vi "Decode and Forward Message.vi"(8 "error in (no error)":errorcluster, 10 "Message undecoded":string, 11 "TCP Listener in":refnum<class "TCP Listener.lvclass">) -> (0 "error out":errorcluster, 3 "TCP Listener out":refnum<class "TCP Listener.lvclass">)   [LabVIEW 2026, in "TALOS.lvlib" / "TCP Listener.lvlib" / "TCP Listener.lvclass"]
uses:
  TCP Listener.lvclass
  C:/LabVIEW Code/TALOS/talos/Father of all uServices/Father of all uServices/Father of all uServices.lvclass
  C:/LabVIEW Code/TALOS/builds/Actor Framework PPL/Actor Framework.lvlibp/1abvi3w/vi.lib/ActorFramework/Actor/Actor.lvclass
  Guardian/Guardian Messages/Message to uService Msg/Message to uService Msg.lvclass/Message to uService Msg.ctl
  Ancestor/Ancestor/Ancestor.lvclass/Ancestor.ctl
  Guardian/Guardian Messages/TCP-SV Message Interpreter Msg/TCP-SV Message Interpreter Msg.lvclass/TCP-SV Message Interpreter Msg.ctl
  Father of all uServices/Father of all uServices/Father of all uServices.lvclass/Father of all uServices.ctl
  TCP Listener.lvclass/TCP Listener.ctl
  Guardian/Guardian Messages/Message to uService Msg/Send Message to uService.vi
  Father of all uServices/Father of all uServices/Children Methods/Update GUI.vi
  Support VIs/Generate Error.vi
  FGV/Error Memory/Get Error Description.vi
  Support VIs/Get PC name.vi
  Ancestor/Ancestor/Read ID.vi
  Support VIs/Get Class Name.vi
  FGV/Error Memory/Error Memory Core.vi
  <vilib>/AdvancedString/Delimited String to 1D String Array.vi
  <vilib>/AdvancedString/Delimited String to 1D String Array (string).vi
  Support VIs/Circus Root Path.vi
  FGV/Error Memory/Error Crt Lvl checker.vi
  FGV/Error Memory/Error Memory Core.vi/40c8088d-b597-4017-91af-faa98e00292e.vi
  FGV/Error Memory/Error Memory Core.vi/d4a3ab98-063c-4e44-b43d-fbdcfe6c2be2.vi
  Father of all uServices/Father of all uServices/Father of all uServices.lvclass
  builds/Actor Framework PPL/Actor Framework.lvlibp/1abvi3w/vi.lib/ActorFramework/Message Enqueuer/Enqueue.vi
  Support VIs/Global Memory.vi
  <vilib>/Utility/LVClass/Get LV Class Name.vi
  Support VIs/Is in Packed Library.vi
  Support VIs/TALOS Root path.vi
  Support VIs/Read CSV worksheet.vi
  Support VIs/Global Constants.vi
  <vilib>/Utility/error.llb/General Error Handler.vi
  Support VIs/Error Log.vi
  Father of all uServices/Father of all uServices/Children Methods/Get GUI Item Value - String.vi
  Father of all uServices/Father of all uServices/Multiline string updater.vi
  Guardian/Guardian Messages/Message to uService Msg/Message to uService Msg.lvclass
  Ancestor/Ancestor/Ancestor.lvclass
  <vilib>/Comparison/Equal/Equal Functor/Equal Functor.lvclass
  Guardian/Guardian Messages/TCP-SV Message Interpreter Msg/TCP-SV Message Interpreter Msg.lvclass
  builds/Actor Framework PPL/Actor Framework.lvlibp/1abvi3w/vi.lib/ActorFramework/Actor/Actor.lvclass
  TALOS.lvlib
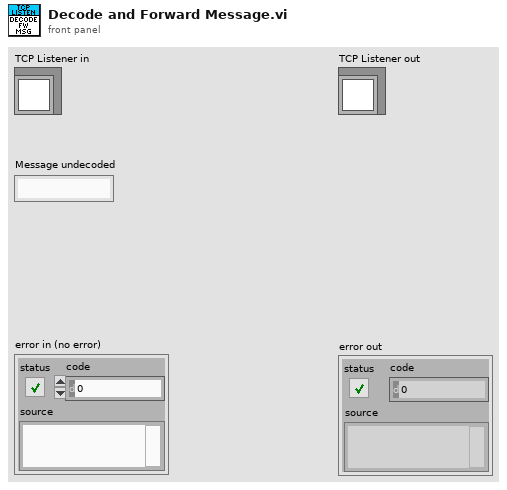
[diagram p1: front panel]
types:
  T1 = typedef "TALOS.lvlib/TCP Writer.lvlib/TCP Writer.lvclass/TCP Message Internal Composition.ctl" = cluster{"uS/GD ID":string, "Message":string, "Data":variant}
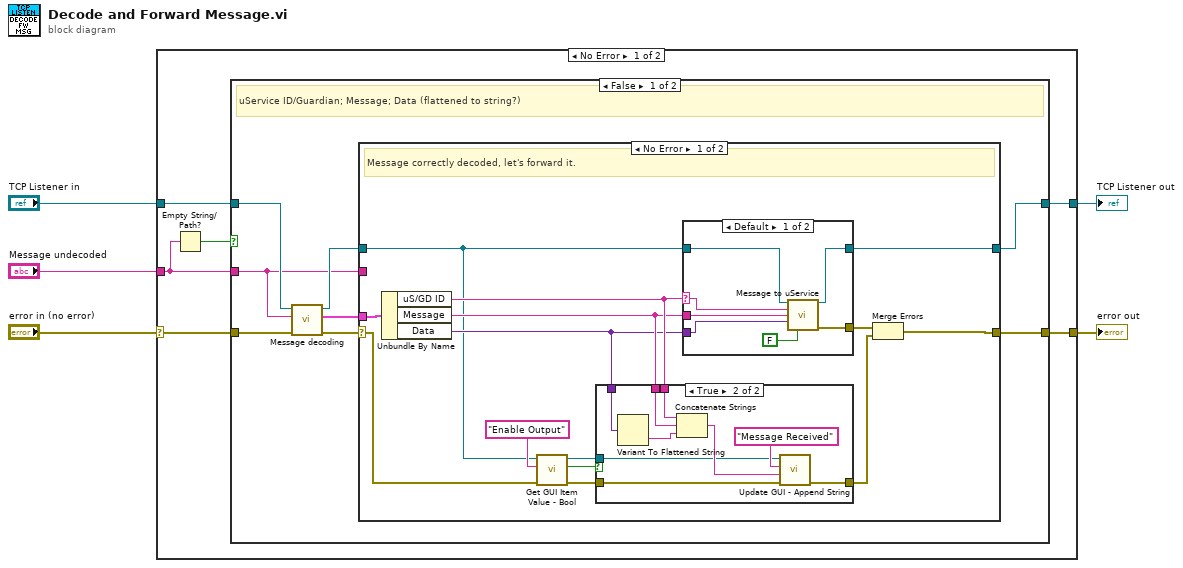
[diagram p0: block diagram]
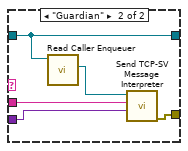
[diagram p3: hidden frame]
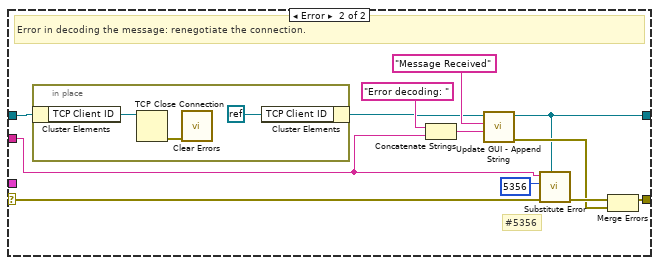
[diagram p4: hidden frame]
diagram:
  n1 = case shown="No Error" "error in (no error)" {
    selector: "error in (no error)" -> [w6 w73]
    tunnel: [w11 w73] -> w5
    tunnel: "TCP Listener in" -> [w10 w74]
    tunnel: [w9 w74] -> w3
    tunnel: "Message undecoded" -> [w8 _]
    frame No Error {
      n2 = Empty String/Path?(string/path=w8) -> (empty?=w7:bool)
      n3 = case shown="False" w7 {
        tunnel: w8 -> [w15 _]
        tunnel: w10 -> [w19 w72]
        tunnel: [w14 w72] -> w9
        tunnel: [w13 w71] -> w11
        tunnel: w6 -> [w12 w71]
        frame False {
          # "uService ID/Guardian; Message; Data (flattened to string?)"
          n4 = call-dynamic "Message decoding.vi"("error in (no error)"=w12, "Message"=w15, "TCP Listener in"=w19) -> ("error out"=w16:errorcluster, "Message decoded"=w18:T1, "TCP Listener out"=w17:refnum<class "TCP Listener.lvclass">)  [unwired: 6 in]
          n5 = case shown="No Error" w16 {
            selector: w16 -> [w24 w67]
            tunnel: w18 -> [w32 _]
            tunnel: [w28 w63] -> w13
            tunnel: w17 -> [w21 w61]
            tunnel: [w26 w56] -> w14
            tunnel: w15 -> [_ w64]
            frame No Error {
              # "Message correctly decoded, let's forward it."
              n6 = Unbundle By Name(w32) -> ("uS/GD ID"=w31:string, "Message"=w30:string, "Data"=w29:variant)
              n7 = call "Get GUI Item Value - Bool.vi"("error in (no error)"=w24, "FP Item Name"="Enable Output" ("Parameter Name"), "uService Template in"=w21) -> ("error out"=w23:errorcluster, "Value"=w22:bool, "uService Template out"=w20:refnum<class "TCP Listener.lvclass">)  [unwired: 6 in]
              n8 = case shown="True" w22 {
                tunnel: w31 -> [_ w41]
                tunnel: w30 -> [_ w40]
                tunnel: w29 -> [_ w39]
                tunnel: [w34 w37] -> w27
                tunnel: w20 -> [_ w36]
                tunnel: w23 -> [w34 w35]
                frame False {
                }
                frame True {
                  n9 = Variant To Flattened String(Variant=w39) -> (data string=w38:string)  [unwired: 1 out]
                  n10 = Concatenate Strings(w41, w40, w38) -> (w42:string)
                  n11 = call "Update GUI - Append String.vi"("error in (no error)"=w35, "String"=w42, "GUI Item Name"="Message Received", "Father of all uServices in"=w36) -> ("error out"=w37:errorcluster)  [unwired: 6 in, 1 out]
                }
              }
              n12 = case shown="Default" w31 {
                selector: w31 -> [w50 _]
                tunnel: w30 -> [w49 w55]
                tunnel: w29 -> [w48 w54]
                tunnel: [w47 w52] -> w33
                tunnel: w21 -> [w46 w51]
                tunnel: [w45 w51] -> w26
                frame Default {
                  n13 = call "Message to uService.vi"("Father of all uServices in"=w46, "uService ID"=w50, "Message"=w49, "Data"=w48, "Locale?"=FALSE) -> ("Father of all uServices out"=w45:refnum<class "TCP Listener.lvclass">, "error out"=w47:errorcluster)  [unwired: 9 in]
                }
                frame "Guardian" {
                  n14 = call "Read Caller Enqueuer.vi"("Actor"=w51) -> ("Caller Enqueuer"=w53:refnum<class "Message Enqueuer.lvclass">)  [unwired: 10 in]
                  n15 = call "Send TCP-SV Message Interpreter.vi"("Data"=w54, "Message"=w55, "Message Enqueuer"=w53) -> ("error out"=w52:errorcluster)  [unwired: 7 in, 1 out]
                }
              }
              n16 = Merge Errors(w33, w27) -> (w28:errorcluster)
            }
            frame Error {
              # "#5356"
              # "Error in decoding the message: renegotiate the connection."
              n17 = in-place {
                n18 = in-place-cluster #1(w61) -> ("TCP Client ID"=w69:refnum<k5>)
                n19 = TCP Close Connection(connection ID=w69) -> (error out=w70:errorcluster)  [unwired: 2 in, 1 out]
                n20 = call <vilib>:"Clear Errors.vi"("error in (no error)"=w70) -> ()  [unwired: 5 in, 2 out]
                n21 = in-place-cluster #1("TCP Client ID"=refnum<k0> refnum) -> (w57:refnum<class "TCP Listener.lvclass">)
              }
              n22 = Concatenate Strings("Error decoding: " ("GUI Item Name"), w64) -> (w58:string)
              n23 = call "Update GUI - Append String.vi"("String"=w58, "GUI Item Name"="Message Received", "Father of all uServices in"=w57) -> ("error out"=w62:errorcluster, "Father of all uServices out"=w56:refnum<class "TCP Listener.lvclass">)  [unwired: 7 in]
              n24 = call "Substitute Error.vi"("LabVIEW Object"=w56, "error in (no error)"=w67, "Error Code"=5356, "Optional String"=w64) -> ("error out"=w66:errorcluster)  [unwired: 7 in]
              n25 = Merge Errors(w66, w62) -> (w63:errorcluster)
            }
          }
        }
        frame True {
          # "Empty string means timeout! Just go back listening."
        }
      }
    }
    frame Error {
    }
  }
  "error out" <- w5
  "TCP Listener out" <- w3
